vi "Read csv.vi"(11 "name or relative path":path) -> (2 "Array 2":dbl[](array[numeric]), 3 "Array":dbl[](array[numeric]))   [LabVIEW 2020]
uses:
  <vilib>/Utility/file.llb/Read Delimited Spreadsheet (DBL).vi
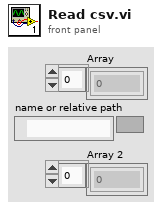
[diagram p1: front panel]
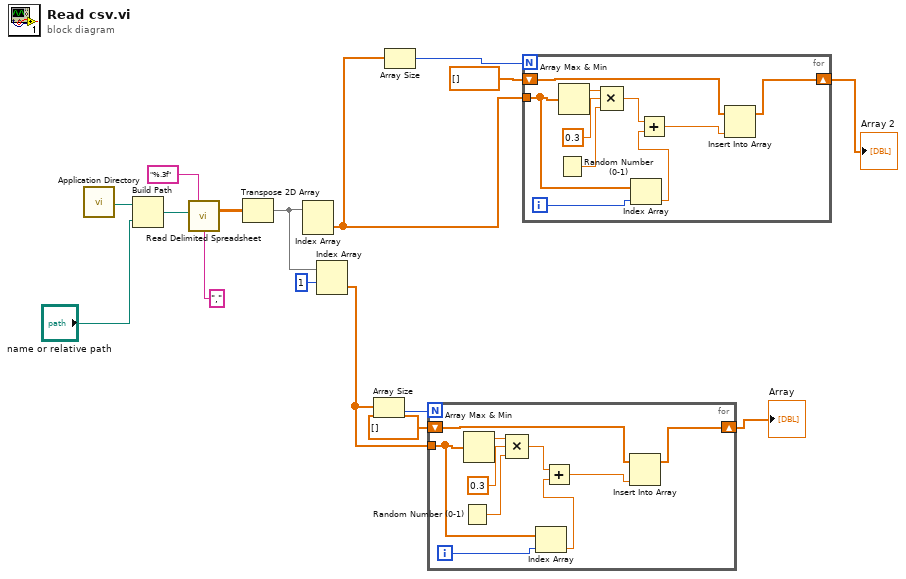
[diagram p0: block diagram]
diagram:
  n1 = call <vilib>:"Application Directory.vi"() -> ("Application Directory"=w10:path)
  n2 = Build Path(base path=w10, name or relative path="name or relative path") -> (appended path=w11:path)
  n3 = call-poly <vilib>:"Read Delimited Spreadsheet.vi"("file path (dialog if empty)"=w11, "format (%.3f)"="%.3f", "delimiter (\\t)"="," ("delimiter (\\t)")) -> ("all rows"=w12:dbl[][])  [unwired: 7 in, 5 out]
  n4 = Transpose 2D Array(2D array=w12) -> (transposed array=w15:dbl[][])
  n5 = Index Array(array=w15) -> (element=w1:dbl[])  [unwired: 2 in]
  n6 = Index Array(array=w15, index (row)=1) -> (element=w7:dbl[])  [unwired: 1 in]
  n7 = Array Size(array=w7) -> (size(s)=w8:i32)
  n8 = Array Size(array=w1) -> (size(s)=w4:i32)
  n9 = for {
    N: w8 -> [_]
    tunnel: w7 -> [w21]
    shift-right: [w19] -> w6
    shift-left: dbl[] [] -> [w18]
    i -> [w22]
    n10 = Random Number (0-1)() -> (number: 0 to 1=w24:dbl)
    n11 = Array Max & Min(array=w21) -> (max value=w25:dbl)  [unwired: 3 out]
    n12 = Compound Arithmetic op=MULTIPLY(w25, 0.3 ("max value"), w24) -> (w26:dbl)
    n13 = Index Array(array=w21, index=w22) -> (element=w20:dbl)
    n14 = Add(x=w26, y=w20) -> (x+y=w17:dbl)
    n15 = Insert Into Array(array=w18, new element=w17) -> (w19:dbl[])  [unwired: 1 in]
  }
  "Array" <- w6
  n16 = for {
    N: w4 -> [_]
    tunnel: w1 -> [w31]
    shift-right: [w29] -> w2
    shift-left: dbl[] [] -> [w28]
    i -> [w32]
    n17 = Random Number (0-1)() -> (number: 0 to 1=w34:dbl)
    n18 = Array Max & Min(array=w31) -> (max value=w35:dbl)  [unwired: 3 out]
    n19 = Compound Arithmetic op=MULTIPLY(w35, 0.3 ("max value"), w34) -> (w36:dbl)
    n20 = Index Array(array=w31, index=w32) -> (element=w30:dbl)
    n21 = Add(x=w36, y=w30) -> (x+y=w27:dbl)
    n22 = Insert Into Array(array=w28, new element=w27) -> (w29:dbl[])  [unwired: 1 in]
  }
  "Array 2" <- w2
